vi "Add Label with Parameters.vi"(8 "error in":errorcluster, 10 "label":T2, 11 "port ref":T1 format="%.0x") -> (0 "error out":errorcluster, 3 "port ref out":T1 format="%.0x")   [LabVIEW 2020, in "AIM ARINC 429 Scripting.lvlib"]
doc: "For Rx labels, this VI assumes SDI, SSM, and Parity have already been added as parameters if desired. For Tx labels, this VI automatically adds trigger channel for acyclic labels or disable channel for scheduled labels."
uses:
  AIM ARINC 429 Scripting.lvlib
  <vilib>/NI VeriStand/Custom Device API/Custom Device Item Ref.ctl
  Shared/VS Channels Definition for Label.ctl
  Shared/VS Channel Definition for Parameter.ctl
  Shared/Parameter Definition.ctl
  <vilib>/NI/NI VeriStand Encoding and Decoding/Encoding.ctl
  Shared/Transfer Type.ctl
  Shared/SDI.ctl
  <vilib>/NI VeriStand/Custom Device API/Custom Device API.lvlib
  <vilib>/NI/NI VeriStand Encoding and Decoding/Encoding and Decoding.lvlib
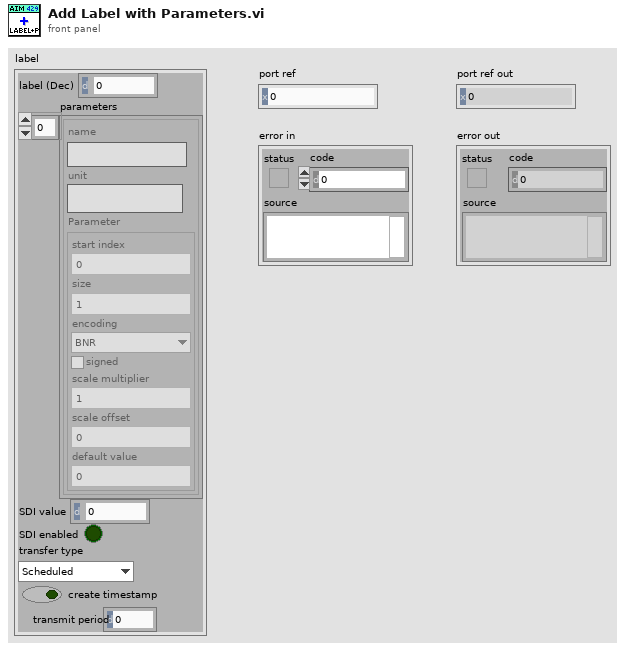
[diagram p1: front panel]
types:
  T1 = typedef "Custom Device API.lvlib/Custom Device Item Ref.ctl" = u64
  T2 = typedef "VS Channels Definition for Label.ctl" = cluster{"label (Dec)":u32, "parameters":T3[], "SDI value":u8, "SDI enabled":bool, "transfer type":T6, "create timestamp":bool, "transmit period":u32}
  T3 = typedef "VS Channel Definition for Parameter.ctl" = cluster{"name":string, "unit":string, "Parameter":T4}
  T4 = typedef "Parameter Definition.ctl" = cluster{"start index":i32, "size":i32, "encoding":T5, "signed":bool, "scale multiplier":dbl, "scale offset":dbl, "default value":dbl}
  T5 = typedef "Encoding and Decoding.lvlib/Encoding.ctl" = enum16{"BNR", "BCD", "Discrete"}
  T6 = typedef "Transfer Type.ctl" = enum16{"Scheduled", "Acyclic", "Block", "Strobe"}
  T7 = typedef "Direction.ctl" = enum16{"Rx", "Tx"}
  T8 = cluster{"SDI":bool, "SSM":bool, "Parity":bool, "Timestamp":bool}
  T9 = typedef "SDI.ctl" = i32
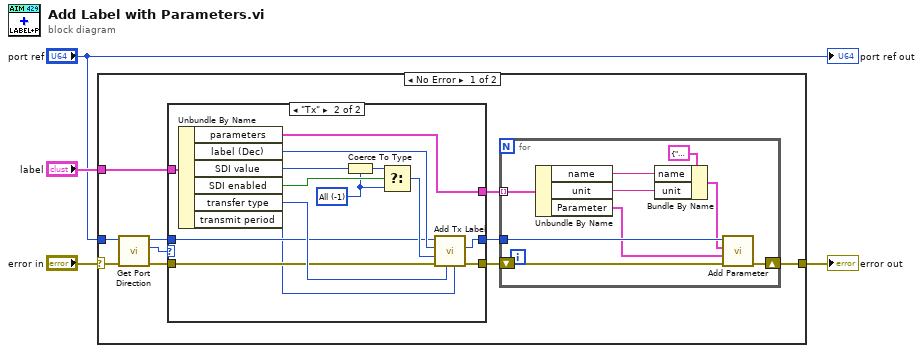
[diagram p0: block diagram]
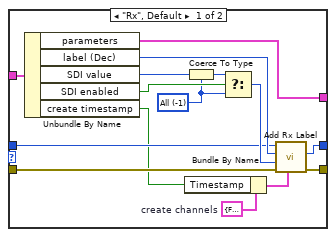
[diagram p2: hidden frame]
diagram:
  n1 = case shown="No Error" "error in" {
    selector: "error in" -> [w9 w53]
    tunnel: "port ref" -> [w7 _]
    tunnel: [w14 w53] -> w4
    tunnel: "label" -> [w13 _]
    frame No Error {
      n2 = call "Get Port Direction.vi"("error in"=w9, "port ref in"=w7) -> ("error out"=w6:errorcluster, "direction"=w5:T7, "port ref out"=w8:T1)  [unwired: 7 in]
      n3 = case shown="\"Tx\"" w5 {
        tunnel: w13 -> [w29 w43]
        tunnel: [w28 w42] -> w12
        tunnel: [w18 w34] -> w11
        tunnel: [w19 w33] -> w10
        tunnel: w8 -> [w21 w32]
        tunnel: w6 -> [w20 w31]
        frame "Rx", Default {
          w17 = T8 {"SDI"=FALSE, "SSM"=FALSE, "Parity"=FALSE, "Timestamp"=FALSE}  # create channels
          w24 = T9 -1 items=["All"=-1, "0 (b00)"=0, "1 (b01)"=1, "2 (b10)"=2, "3 (b11)"=3] ("SDI value")
          n4 = Unbundle By Name(w29) -> ("parameters"=w28:T3[], "label (Dec)"=w22:u32, "SDI value"=w26:u8, "SDI enabled"=w27:bool, "create timestamp"=w16:bool)
          n5 = Bundle By Name(cluster=w17, "Timestamp"=w16) -> (w15:T8)
          n6 = Coerce To Type(0:w26, 1:w24) -> (2:w25:T9)
          n7 = Select(t=w25, s=w27, f=w24) -> (s? t:f=w23:T9)
          n8 = call "Add Rx Label.vi"("create channels"=w15, "error in"=w20, "SDI value"=w23, "label value"=w22, "port in"=w21) -> ("error out"=w18:errorcluster, "label"=w19:T1)  [unwired: 4 in, 1 out]
        }
        frame "Tx" {
          w38 = T9 -1 items=["All"=-1, "0 (b00)"=0, "1 (b01)"=1, "2 (b10)"=2, "3 (b11)"=3] ("SDI value")
          n9 = Unbundle By Name(w43) -> ("parameters"=w42:T3[], "label (Dec)"=w35:u32, "SDI value"=w40:u8, "SDI enabled"=w41:bool, "transfer type"=w36:T6, "transmit period"=w30:u32)
          n10 = Coerce To Type(0:w40, 1:w38) -> (2:w39:T9)
          n11 = Select(t=w39, s=w41, f=w38) -> (s? t:f=w37:T9)
          n12 = call "Add Tx Label.vi"("scheduled transmit period (us)"=w30, "transfer type"=w36, "error in"=w31, "SDI value"=w37, "label value"=w35, "port in"=w32) -> ("error out"=w34:errorcluster, "label"=w33:T1)  [unwired: 3 in, 1 out]
        }
      }
      n13 = for {
        shift-right: [w50] -> w14
        shift-left: w11 -> [w51]
        tunnel: w12 -> [w49] mode=indexing
        tunnel: w10 -> [w52]
        n14 = Unbundle By Name(w49) -> ("name"=w46:string, "unit"=w45:string, "Parameter"=w48:T4)
        n15 = Bundle By Name(cluster=cluster{"name":string, "unit":string} {"name"="", "unit"=""} ("parameter"), "name"=w46, "unit"=w45) -> (w44:cluster{"name":string, "unit":string})
        n16 = call "Add Parameter.vi"("error in"=w51, "parameter encoding"=w48, "parameter definition"=w44, "label in"=w52) -> ("error out"=w50:errorcluster)  [unwired: 5 in, 2 out]
      }
    }
    frame Error {
    }
  }
  "error out" <- w4
  "port ref out" <- "port ref"
